vi "test_IntrinsicImagingMG091001.vi"() -> ()   [LabVIEW 2010, in "DataCollectionMG091001IntrinsicImaging.lvclass"]
uses:
  DataCollectionMG091001IntrinsicImaging.lvclass
  common/classes/Image/Image/Image.lvclass
  main/labview_source/type_definitions/clusters/controls_refs.ctl
  common/classes/GenericToplevelComponent/GenericToplevelComponent/common_trigger_enum.ctl
  GenericDataCollection/GenericDataCollection/GenericDataCollection.lvclass
  GenericDataCollection/GenericDataCollection/trigger_enum.ctl
  common/classes/GenericToplevelComponent/GenericToplevelComponent/GenericToplevelComponent.lvclass
panel:
  in  "brighten stimulation":dbl=1.0
  in  "save button":bool
  in  "number of sweeps":i32=4
  in  "stimulation only?":bool
  in  "sendButton":bool
  out "done?":bool
  in  "reset":bool
  in  "phase offset duration":dbl[unit]
  in  "phase duration":dbl[unit]=1.0
  in  "runButton":bool
  in  "stop":bool
  in  "loadButton":bool
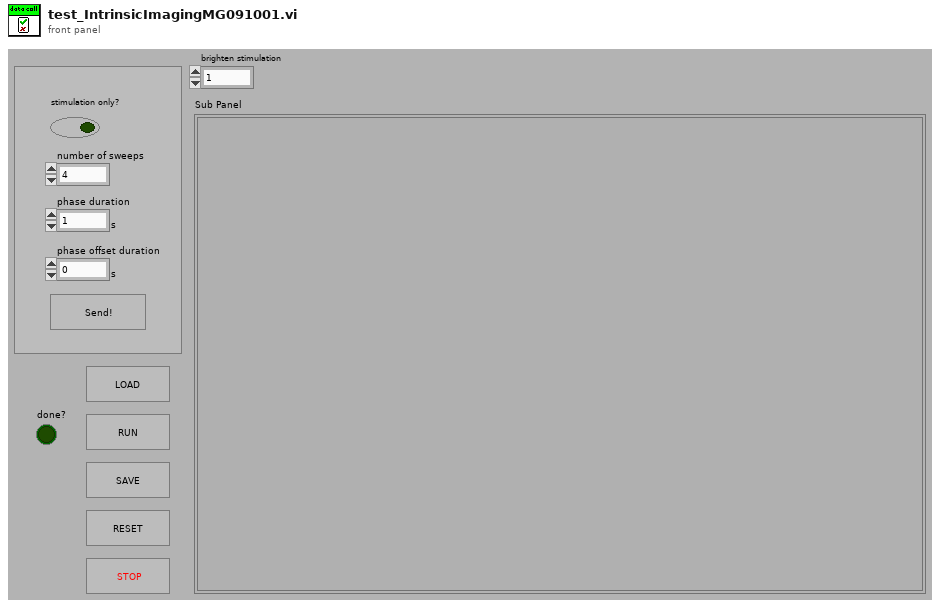
[diagram p1: front panel]
types:
  T1 = typedef "controls_refs.ctl" = cluster{"scan start button":refnum<vi>, "tabs":cluster{"main":refnum<vi>, "settings":refnum<vi>}, "subpanels":cluster{"imagingMode":refnum<vi>, "scanHead":refnum<vi>, "display":refnum<vi>, "experimentController":refnum<vi>, "instrument":refnum<vi>, "stage":refnum<vi>, "stimulator":refnum<vi>, "dataCollection":refnum<vi>, "analyser":refnum<vi>, "daq":refnum<vi>, "imageAssembler":refnum<vi>}, "drop-downs":cluster{"run mode":refnum<vi>, "imagingMode":refnum<vi>, "experimentalController":refnum<vi>, "objective":refnum<vi>}, "status lights":cluster{"experimentController":refnum<vi>, "imagingMode":refnum<vi>, "scanHead":refnum<vi>, "daq":refnum<vi>, "imageAssembler":refnum<vi>, "dataCollection":refnum<vi>, "display":refnum<vi>, "analyser":refnum<vi>, "stage":refnum<vi>, "stimulator":refnum<vi>, "instrument":refnum<vi>}, "message":refnum<vi>, "stimulator enabled?":refnum<vi>, "saving":cluster{"data folder path":refnum<vi>, "file base name":refnum<vi>, "notebook":refnum<vi>}, "progress bar":refnum<vi>, "update icon":refnum<vi>, "title":refnum<vi>, "main vi":refnum<vi>, "user":refnum<vi>, "exit_button":refnum<vi>, "CPU usage %":refnum<vi>}
  T2 = typedef "GenericToplevelComponent.lvclass/common_trigger_enum.ctl" = enum16{"NULL", "initialise", "terminate", "fetch command", "fetch data", "attach observer", "register as observer", "detach observer", "acknowledge", "start", "stop"}
  T3 = typedef "GenericDataCollection.lvclass/trigger_enum.ctl" = enum16{"NULL", "save"}
  T4 = typedef "Image Type" = u32
  T5 = typedef "plugin_specification.ctl" = cluster{"class path":string, "configuration":string, "label":string, "settings name":string}
  T6 = typedef "XComponentSpecification.xctl/data.ctl" = cluster{"class path":string, "configuration":string, "label":string, "settings name":string}
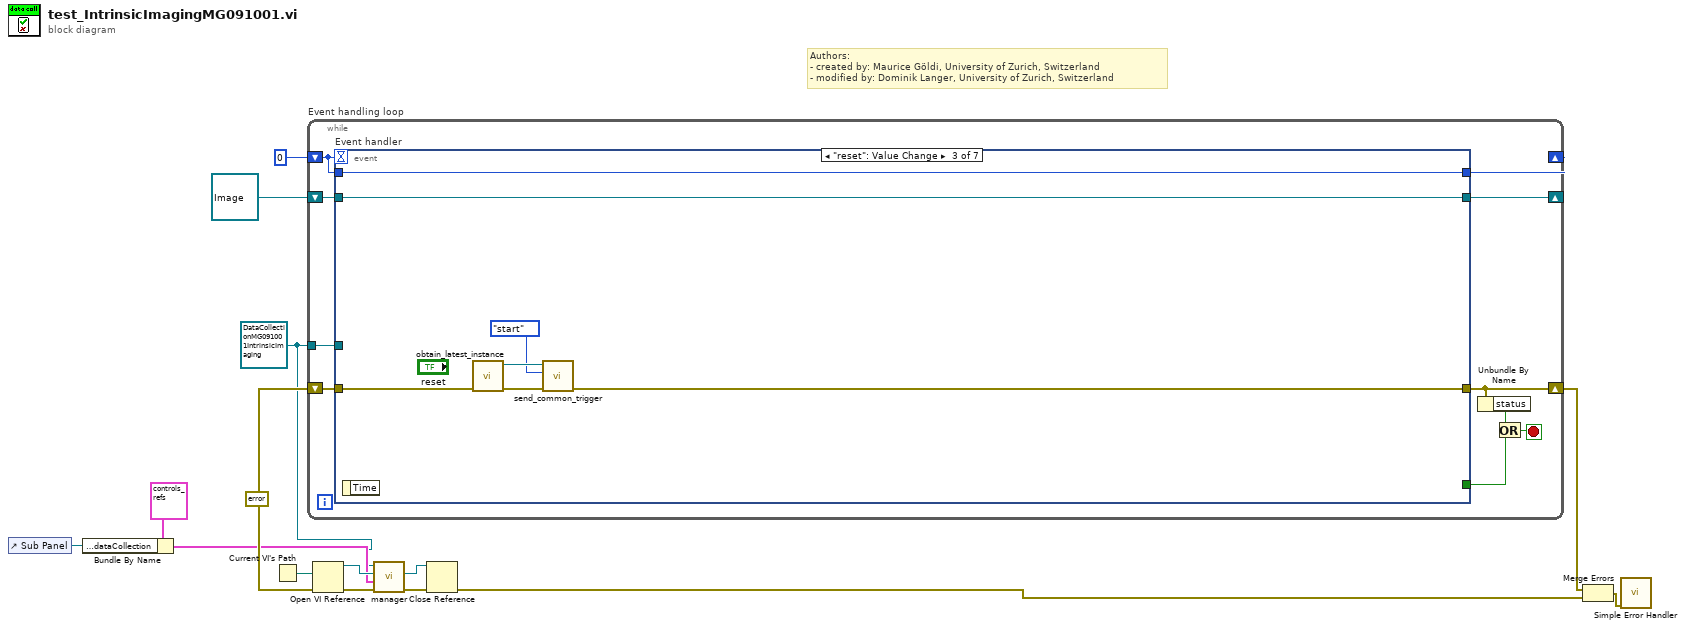
[diagram p0: block diagram]
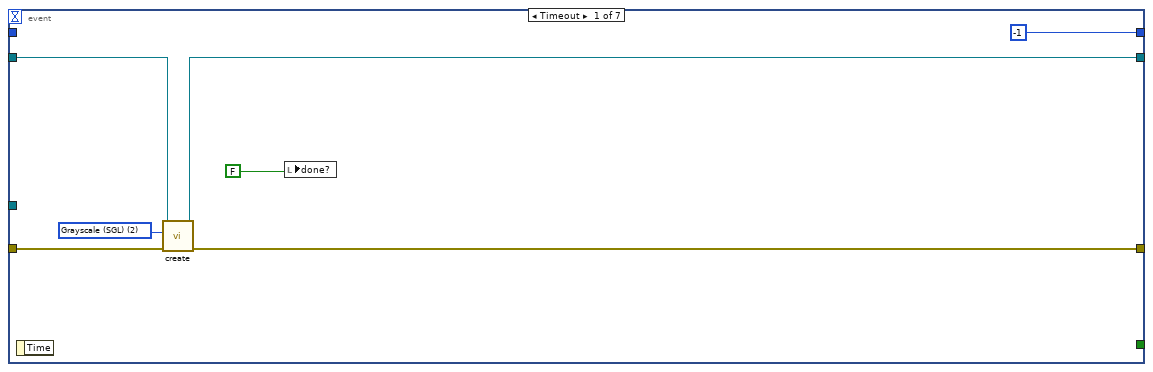
[diagram p2: hidden frame]
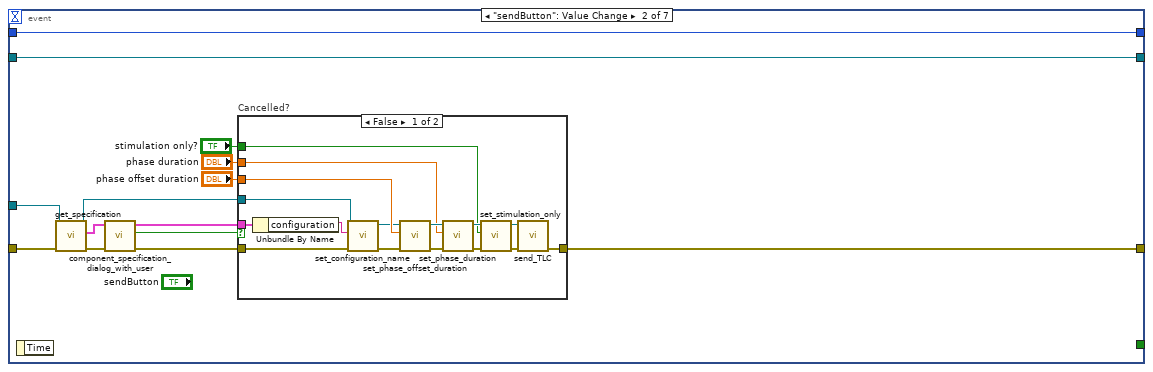
[diagram p3: hidden frame]
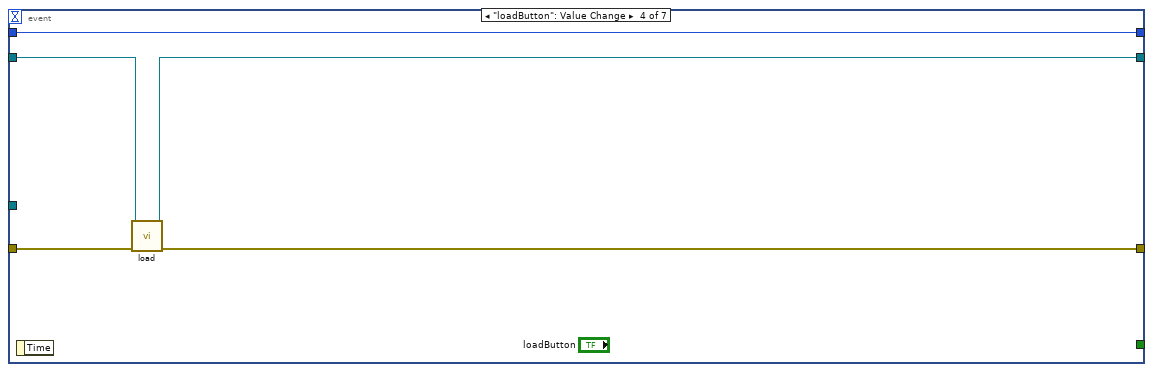
[diagram p5: hidden frame]
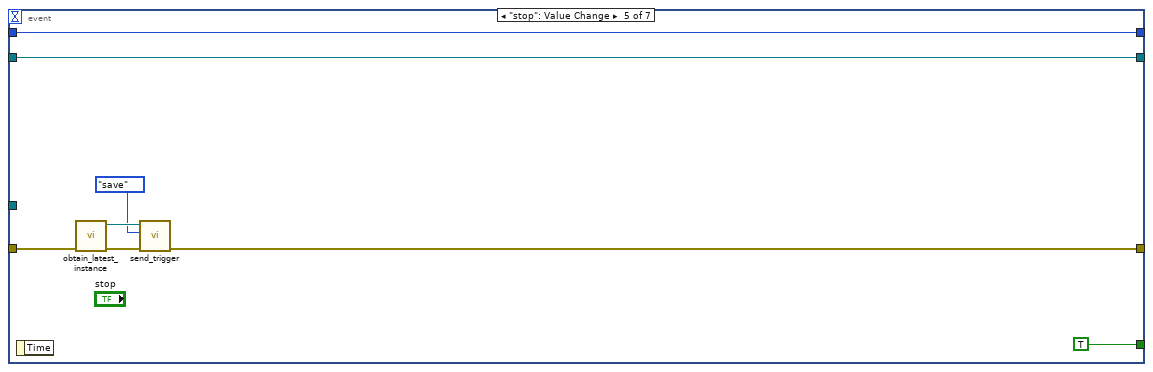
[diagram p6: hidden frame]
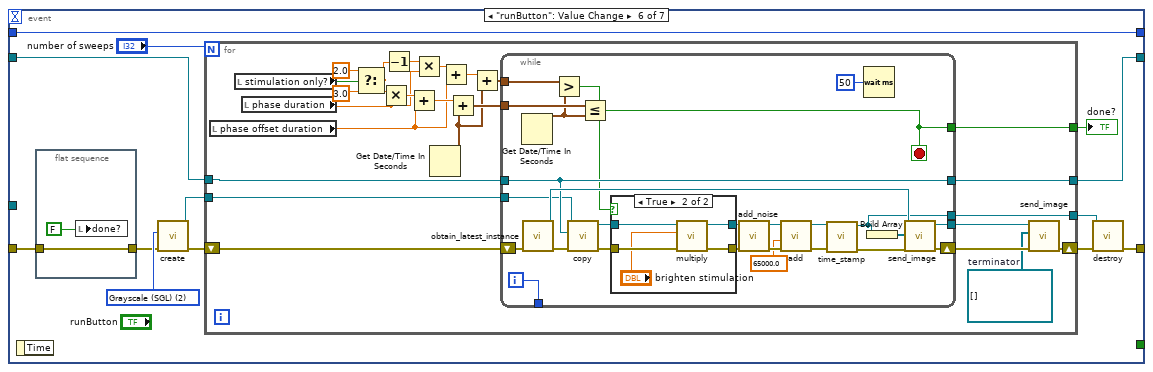
[diagram p7: hidden frame]
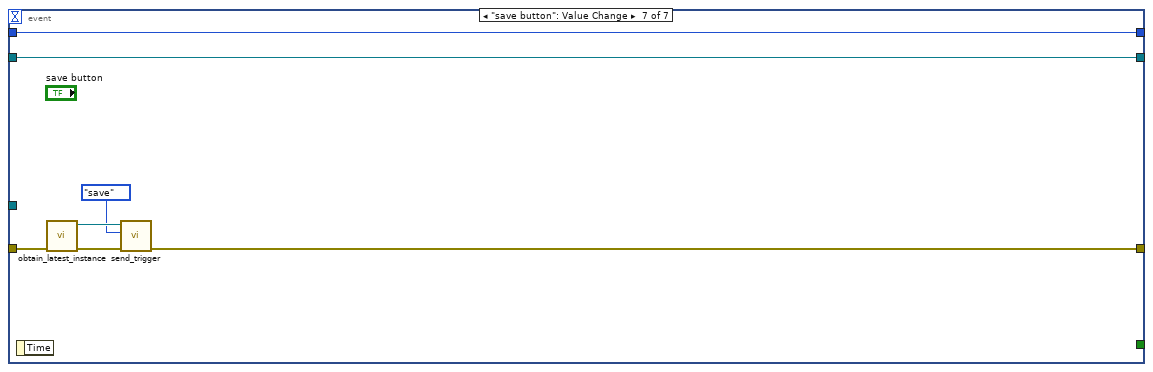
[diagram p9: hidden frame]
diagram:
  w1 = refnum<class "DataCollectionMG091001IntrinsicImaging.lvclass"> refnum ("IntrinsicImagingMG091001.lvclass")
  w11 = errorcluster {"status"=FALSE, "code"=0, "source"=""} ("error out")
  # "Authors: \n- created by: Maurice Göldi, University of Zurich, Switzerland\n- modified by: Dominik Langer, University of Zurich, Switzerland"
  n1 = control-ref of="Sub Panel"() -> (w2:refnum<vi>)
  n2 = Bundle By Name(cluster=T1 {"scan start button"=refnum, "tabs"={"main"=refnum, "settings"=refnum}, "subpanels"={"imagingMode"=refnum, "scanHead"=refnum, "display"=refnum, "experimentController"=refnum, "instrument"=refnum, "stage"=refnum, "stimulator"=refnum, "dataCollection"=refnum, "analyser"=refnum, "daq"=refnum, "imageAssembler"=refnum}, "drop-downs"={"run mode"=refnum, "imagingMode"=refnum, "experimentalController"=refnum, "objective"=refnum}, "status lights"={"experimentController"=refnum, "imagingMode"=refnum, "scanHead"=refnum, "daq"=refnum, "imageAssembler"=refnum, "dataCollection"=refnum, "display"=refnum, "analyser"=refnum, "stage"=refnum, "stimulator"=refnum, "instrument"=refnum}, "message"=refnum, "stimulator enabled?"=refnum, "saving"={"data folder path"=refnum, "file base name"=refnum, "notebook"=refnum}, "progress bar"=refnum, "update icon"=refnum, "title"=refnum, "main vi"=refnum, "user"=refnum, "exit_button"=refnum, "CPU usage %"=refnum} ("control references"), "subpanels.dataCollection"=w2) -> (w3:T1)
  n3 = Current VI's Path() -> (path=w5:path)
  n4 = while "Event handling loop" {
    shift-right: [w20] -> w14
    shift-left: w11 -> [w24]
    shift-right: [w21] -> _
    shift-left: 0 -> [w25]
    shift-right: [w22] -> _
    shift-left: refnum<class "Image.lvclass"> refnum ("Image.lvclass") -> [w23]
    tunnel: w1 -> [w16]
    stop <- w17 stop-if-true
    n5 = event "Event handler" shown="[2] \"reset\": Value Change" {
      selector: _ -> [_ _ _ _ _ _ _]
      dyn-events: _ -> [_ _ _ _ _ _ _]
      timeout: w25 -> [_ _ _ _ _ _ _]
      tunnel: [-1 w46 w70 w75 w83 w95 w162] -> w21
      tunnel: w25 -> [_ w46 w70 w75 w83 w95 w162]
      tunnel: w24 -> [w30 w38 w67 w74 w79 w86 w159]
      tunnel: [w26 w42 w66 w73 w78 w91 w158] -> w20
      tunnel: w23 -> [w29 w45 w69 w72 w81 w96 w161]
      tunnel: [w28 w45 w69 w71 w81 w94 w161] -> w22
      tunnel: [_ _ _ _ TRUE _ _] -> w18
      tunnel: w16 -> [_ w40 _ _ _ _ _]
      event Timeout {
        w31 = T4 2 items=["Grayscale (U8)", "Grayscale (I16)", "Grayscale (SGL)", "Complex (CSG)", "RGB (U32)", "HSL (U32)", "RGB (U64)", "Grayscale (U16)"] ("Image Type")
        n6 = event-data() -> ()  [unwired: 1 in, 1 out]
        n7 = call "create.vi"("error in (no error)"=w30, "Image Type"=w31, "Image in"=w29) -> ("error out"=w26:errorcluster, "Image out"=w28:refnum<class "Image.lvclass">)  [unwired: 7 in]
        n8 = local write "done?"(FALSE) -> ()
      }
      event "sendButton": Value Change {
        n9 = event-data() -> ()  [unwired: 1 in, 1 out]
        n10 = call-dynamic "get_specification.vi"("error in (no error)"=w38, "GenericPlugin in"=w40) -> ("error out"=w37:errorcluster, "component specification"=w39:T5, "GenericPlugin out"=w33:refnum<class "DataCollectionMG091001IntrinsicImaging.lvclass">)  [unwired: 6 in, 1 out]
        n11 = call "component_specification_dialog_with_user.vi"("error in (no error)"=w37, "component specification in"=w39) -> ("error out"=w36:errorcluster, "cancelled?"=w35:bool, "component specification out"=w34:T6)  [unwired: 7 in]
        n12 = case "Cancelled?" shown="False" w35 {
          tunnel: "phase offset duration" -> [w58 _]
          tunnel: "phase duration" -> [w57 _]
          tunnel: [w56 w63] -> w42
          tunnel: "stimulation only?" -> [w55 _]
          tunnel: w36 -> [w50 w63]
          tunnel: w34 -> [w49 _]
          tunnel: w33 -> [w48 _]
          frame False {
            n13 = Unbundle By Name(w49) -> ("configuration"=w47:string)
            n14 = call-dynamic "set_configuration_name.vi"("error in (no error)"=w50, "configuration"=w47, "GenericPlugin.lvclass in"=w48) -> ("error out"=w52:errorcluster, "GenericPlugin.lvclass out"=w51:refnum<class "DataCollectionMG091001IntrinsicImaging.lvclass">)  [unwired: 7 in]
            n15 = call "set_phase_offset_duration.vi"("error in (no error)"=w52, "phase offset duration"=w58, "IntrinsicImagingMG091001 in"=w51) -> ("error out"=w62:errorcluster, "IntrinsicImagingMG091001 out"=w60:refnum<class "DataCollectionMG091001IntrinsicImaging.lvclass">)  [unwired: 7 in]
            n16 = call "set_phase_duration.vi"("error in (no error)"=w62, "phase duration"=w57, "IntrinsicImagingMG091001 in"=w60) -> ("error out"=w61:errorcluster, "IntrinsicImagingMG091001 out"=w59:refnum<class "DataCollectionMG091001IntrinsicImaging.lvclass">)  [unwired: 7 in]
            n17 = call-dynamic "set_stimulation_only.vi"("error in (no error)"=w61, "stimulation only?"=w55, "IntrinsicImagingMG091001 in"=w59) -> ("error out"=w54:errorcluster, "IntrinsicImagingMG091001 out"=w53:refnum<class "DataCollectionMG091001IntrinsicImaging.lvclass">)  [unwired: 7 in]
            n18 = call-dynamic "send_TLC.vi"("error in (no error)"=w54, "GenericToplevelComponent in"=w53) -> ("error out"=w56:errorcluster)  [unwired: 8 in, 1 out]
          }
          frame True {
          }
        }
      }
      event "reset": Value Change {
        n19 = event-data() -> ()  [unwired: 1 in, 1 out]
        n20 = call "obtain_latest_instance.vi"("error in (no error)"=w67) -> ("error out"=w68:errorcluster, "GenericDataCollection out"=w65:refnum<class "GenericDataCollection.lvclass">)  [unwired: 9 in]
        n21 = call-dynamic "send_common_trigger.vi"("error in (no error)"=w68, "trigger"=common_trigger_enum."start", "GenericToplevelComponent in"=w65) -> ("error out"=w66:errorcluster)  [unwired: 6 in, 2 out]
      }
      event "loadButton": Value Change {
        n22 = event-data() -> ()  [unwired: 1 in, 1 out]
        n23 = call-dynamic "load.vi"("error in (no error)"=w74, "Image in"=w72) -> ("error out"=w73:errorcluster, "Image out"=w71:refnum<class "Image.lvclass">)  [unwired: 6 in, 2 out]
      }
      event "stop": Value Change {
        n24 = event-data() -> ()  [unwired: 1 in, 1 out]
        n25 = call "obtain_latest_instance.vi"("error in (no error)"=w79) -> ("error out"=w80:errorcluster, "GenericDataCollection out"=w77:refnum<class "GenericDataCollection.lvclass">)  [unwired: 9 in]
        n26 = call-dynamic "send_trigger.vi"("error in (no error)"=w80, "trigger"=trigger_enum."save", "GenericDataCollection in"=w77) -> ("error out"=w78:errorcluster)  [unwired: 7 in, 1 out]
      }
      event "runButton": Value Change {
        w89 = T4 2 items=["Grayscale (U8)", "Grayscale (I16)", "Grayscale (SGL)", "Complex (CSG)", "RGB (U32)", "HSL (U32)", "RGB (U64)", "Grayscale (U16)"] ("Image Type")
        n27 = event-data() -> ()  [unwired: 1 in, 1 out]
        n28 = flat-sequence {
          tunnel: w86 -> [w155]
          tunnel: [w155] -> w85
          frame #0 {
            n29 = local write "done?"(FALSE) -> ()
          }
        }
        n30 = call "create.vi"("error in (no error)"=w85, "Image Type"=w89) -> ("error out"=w93:errorcluster, "Image out"=w92:refnum<class "Image.lvclass">)  [unwired: 8 in]
        n31 = for {
          N: "number of sweeps" -> [_]
          tunnel: w96 -> [w120]
          tunnel: [w117] -> w94
          tunnel: w92 -> [w115]
          tunnel: [w114] -> w90
          tunnel: [w105] -> w87
          shift-right: [w108] -> w88
          shift-left: w93 -> [w116]
          w106 = refnum<class "Image.lvclass">[] []  # terminator
          n32 = local read "phase offset duration"() -> (w100:dbl[unit])
          n33 = local read "stimulation only?"() -> (w113:bool)
          n34 = local read "phase duration"() -> (w102:dbl[unit])
          n35 = Select(t=2.0, s=w113, f=3.0) -> (s? t:f=w104:dbl)
          n36 = Multiply(x=w104, y=w102) -> (x*y=w119:dbl[unit])
          n37 = Decrement(x=w104) -> (x-1=w103:dbl)
          n38 = Add(x=w119, y=w100) -> (x+y=w110:dbl[unit])
          n39 = Multiply(x=w103, y=w102) -> (x*y=w101:dbl[unit])
          n40 = Get Date/Time In Seconds() -> (seconds since 1Jan1904=w99:timestamp)
          n41 = Add(x=w101, y=w100) -> (x+y=w98:dbl[unit])
          n42 = Add(x=w110, y=w99) -> (x+y=w118:timestamp)
          n43 = Add(x=w98, y=w99) -> (x+y=w97:timestamp)
          n44 = while {
            shift-right: [w137] -> w109
            shift-left: w116 -> [w142]
            tunnel: w118 -> [w144]
            tunnel: w120 -> [w140]
            tunnel: [w140] -> w117
            tunnel: w115 -> [w138]
            tunnel: [w136] -> w114
            tunnel: [w135] -> w107
            tunnel: [w134] -> w105
            tunnel: [w133] -> _
            tunnel: w97 -> [w130]
            i -> [w133]
            stop <- w134 stop-if-true
            n45 = Get Date/Time In Seconds() -> (seconds since 1Jan1904=w129:timestamp)
            n46 = call "obtain_latest_instance.vi"("error in (no error)"=w142) -> ("error out"=w139:errorcluster, "GenericDataCollection out"=w141:refnum<class "GenericDataCollection.lvclass">)  [unwired: 9 in]
            n47 = Greater?(x=w130, y=w129) -> (0:w128:bool)
            n48 = call "copy.vi"("error in (no error)"=w139, "image to copy (source)"=w140, "Image in (target)"=w138) -> ("error out"=w127:errorcluster, "Image out"=w126:refnum<class "Image.lvclass">)  [unwired: 7 in]
            n49 = Less Or Equal?(x=w144, y=w129) -> (x <= y?=w134:bool)
            n50 = case shown="True" w128 {
              tunnel: w127 -> [w147 w153]
              tunnel: [w147 w152] -> w132
              tunnel: w126 -> [w148 w151]
              tunnel: [w148 w150] -> w131
              frame False {
              }
              frame True {
                n51 = call-dynamic "multiply.vi"("error in (no error)"=w153, "factor"="brighten stimulation", "Image in"=w151) -> ("error out"=w152:errorcluster, "Image out"=w150:refnum<class "Image.lvclass">)  [unwired: 7 in]
              }
            }
            n52 = call "add_noise.vi"("error in (no error)"=w132, "Image in"=w131) -> ("error out"=w125:errorcluster, "Image out"=w123:refnum<class "Image.lvclass">)  [unwired: 8 in]
            n53 = call-dynamic "add.vi"("error in (no error)"=w125, "constant"=sgl 65000.0, "Image in"=w123) -> ("error out"=w124:errorcluster, "Image out"=w122:refnum<class "Image.lvclass">)  [unwired: 7 in]
            n54 = call-dynamic "time_stamp.vi"("error in (no error)"=w124, "Image in"=w122) -> ("error out"=w146:errorcluster, "Image out"=w136:refnum<class "Image.lvclass">)  [unwired: 8 in]
            n55 = Wait (ms)(milliseconds to wait=u32 50) -> ()  [unwired: 1 out]
            n56 = Build Array(w136) -> (w145:refnum<class "Image.lvclass">[])
            n57 = call-dynamic "send_image.vi"("error in (no error)"=w146, "image (channels)"=w145, "GenericToplevelComponent in"=w141) -> ("error out"=w137:errorcluster, "GenericToplevelComponent out"=w135:refnum<class "GenericDataCollection.lvclass">)  [unwired: 6 in, 1 out]
          }
          n58 = call-dynamic "send_image.vi"("error in (no error)"=w109, "image (channels)"=w106, "GenericToplevelComponent in"=w107) -> ("error out"=w108:errorcluster)  [unwired: 6 in, 2 out]
        }
        "done?" <- w87
        n59 = call-dynamic "destroy.vi"("error in (no error)"=w88, "Image in"=w90) -> ("error out"=w91:errorcluster)  [unwired: 8 in, 1 out]
      }
      event "save button": Value Change {
        n60 = event-data() -> ()  [unwired: 1 in, 1 out]
        n61 = call "obtain_latest_instance.vi"("error in (no error)"=w159) -> ("error out"=w160:errorcluster, "GenericDataCollection out"=w157:refnum<class "GenericDataCollection.lvclass">)  [unwired: 9 in]
        n62 = call-dynamic "send_trigger.vi"("error in (no error)"=w160, "trigger"=trigger_enum."save", "GenericDataCollection in"=w157) -> ("error out"=w158:errorcluster)  [unwired: 7 in, 1 out]
      }
    }
    n63 = Unbundle By Name(w20) -> ("status"=w19:bool)
    n64 = Or(x=w19, y=w18) -> (x .or. y?=w17:bool)
  }
  n65 = Open VI Reference(vi path=w5, error in (no error)=w11) -> (vi reference=w6:refnum<vi>, error out=w10:errorcluster)  [unwired: 4 in]
  n66 = call-dynamic "manager.vi"("error in (no error)"=w10, "control references"=w3, "top-level VI ref in"=w6, "GenericToplevelComponent in"=w1) -> ("error out"=w9:errorcluster, "top-level VI ref out"=w7:refnum<vi>)  [unwired: 5 in, 1 out]
  n67 = Close Reference(reference=w7, error in (no error)=w9) -> (error out=w8:errorcluster)
  n68 = Merge Errors(w14, w8) -> (w15:errorcluster)
  n69 = call <vilib>:"Simple Error Handler.vi"("error in (no error)"=w15) -> ()  [unwired: 4 in, 5 out]
